vi "信号光谱2.vi"() -> ()   [LabVIEW 2015]
uses:
  <vilib>/Utility/file.llb/Write Delimited Spreadsheet (DBL).vi
  <vilib>/Analysis/NI_AALBase.lvlib
panel:
  out "最终存储路径":path
  in  "停止程序":bool
  in  "上升下降沿/s":dbl format="%.2p"
  in  "延时/s":dbl format="%.2p"
  in  "占空比/%":dbl=3.0 format="%.2p"
  in  "高电平/V":dbl=4.0 format="%.2p"
  in  "频率/Hz":dbl=100.0 format="%.3p"
  in  "低电平/V":dbl min=0.0 max=5.0 format="%.2p"
  out "configure error out":errorcluster
  in  "设置参数":bool
  out "output control error  4":errorcluster
  in  "低电平持续输出":bool
  in  "Output 1":bool
  out "output control error  5":errorcluster
  in  "脉冲作用时间/s":dbl=1.0
  in  "测量高电平/V":dbl=4.0
  out "output control error  2":errorcluster
  in  "测量次数":i32=1
  in  "开始测量":bool
  in  "上升下降沿":i32(ring)=1 items=["上升沿", "下降沿"]
  in  "channel输出口":i32(ring) items=["Channel 1", "Channel 2"]
  in  "输出信号波形":u16(ring) items=["Pulse"]
  out "output control error  3":errorcluster
  out "Output":bool
  in  "VISA 信号发生器":refnum<visa-resource-name>="USB0::0x1AB1::0x0641::DG4E192200870::INSTR"
  out "Spectrum":cluster{"Y":dbl[], "Y":dbl[]}[](graph)
  in  "计数器":dbl=720.0
  out "波长范围":dbl[](array[numeric])
  in  "选项卡控件":enum32{"IHR 550", "CCD"}(tab)
  in  "Move To\nTarget Positions":bool
  out "Current UniqueID":string="Mono4"
  in  "Mono ID":string(combo)="Mono1"
  in  "Connect":bool
  out "Initialized JY":bool=TRUE
  in  "Force\nInitialization":bool
  in  "Target Grating":string(combo)="2"
  out "Current Description":string="1" caption="Description"
  out "Grating Index":i32=1
  out "Current Grating":dbl=1200.0
  out "Units":string="nm"
  out "Current WL":dbl=897.9988
  out "Exit Mirror\nPosition":i32(ring)=2 items=["EntranceMirror", "ExitMirror", "Front", "Side"]
  out "Entrance Mirror\nPosition":i32(ring)=2 items=["EntranceMirror", "ExitMirror", "Front", "Side"]
  out "Units 2":string="mm"
  out "Front Entrance":dbl
  in  "Target WL":dbl=2670.0
  in  "Exit Mirror":u16(ring)=3 caption="Target Position Exit Mirror" items=["Front"=2, "Side"=3]
  in  "Entrance Mirror":u16(ring)=2 caption="Target Position\nEntrance Mirror" items=["Front"=2, "Side"=3]
  in  "Target\nFront Entrance":dbl=1.0
  in  "Commande tab":T1(tab)
  in  "Area Number to Display":i32
  in  "Reformat":bool
  in  "GAIN":u16(ring)=2 caption="Device Name" items=["High Light", "Best Dynamic Range", "High Sensitivity"]
  in  "ADC":u16(ring) caption="Device Name" items=["20 kHz       ", " 1 MHz       ", " 1 MHz Ultra "]
  in  "Number of Areas :":u16=1 min=1 step=1
  in  "Integration time (ms) :":i32=5000
  out "Uniques ID":u16(ring) items=["CCD1", "CCD2"]
  in  "Device Name":u16(ring) items=["Synapse CCD (Lateral)", "Synapse_IGA (Axial)"]
  in  "Signal type :":enum16{"TTL Rising Edge", "TTL Falling Edge"}(ring)=enum."TTL Falling Edge"
  in  "Trigger Type :":u16(ring) items=["On Start"=1, "Per Acquisition"=2]
  in  "trigSigTypeString":string
  in  "trigEventString":string
  in  "Enable InputTriggers :":bool
  in  "Number of Cleans":i32=1
  in  "MultiAcqShutterMode":i32(ring)=3 items=["Open For All Spectra"=1, "Open for Each Spectrum"=3]
  in  "Accumulations:":u16=10 min=1 step=1
  in  "Multi Accumulation mode:":bool
  out "Y Pixels:":i32=256
  out "DataSize":i32=1024
  out "X Pixels:":i32=1024
  out "Firmware\nVersion":string="V1.20 CCD_4000"
  out "initialized ?":bool=TRUE
  in  "Continuous":bool
  in  "CCD Busy":bool
  out "indicator":string="Ready !"
  in  "initialize":bool
  in  "ShutterOpen":bool=TRUE caption="Shutter enable"
  in  "Save Backlight":bool
  in  "Acquire":bool
  in  "Temperature":bool
  in  "Setup":bool
  in  "起始波长":dbl=2406.79
  in  "终止波长":dbl=2919.91
  out "Acq Time(ms)":u32=3401
  in  "Close":bool=TRUE
  out "JYCCDLib.IJYCCDReqd":refnum<k7>
  out "areas :":i32[][](array[numeric])=[[1], [1], [1], [1024], [256], [1], [256]]
  in  "Constante de condition\n(Voir l'aide contextuelle)":bool
  out "temp graph":dbl(graph)=-134.538067
  out "ADC Number":i32[](array[numeric])=[0, 1, 2, 3, 4]
  out "Gain Number":i32[](array[numeric])=[10, 11, 12, 13, 8, 2]
  out "trigAddress":i32
  out "Data":i32[][](graph)
  out "error out":errorcluster
  out "Gratings":dbl[](array[numeric])=[1200.0, 300.0]
  out "Backlight":i32[][](graph)
  out "data 2":i32[][](graph)
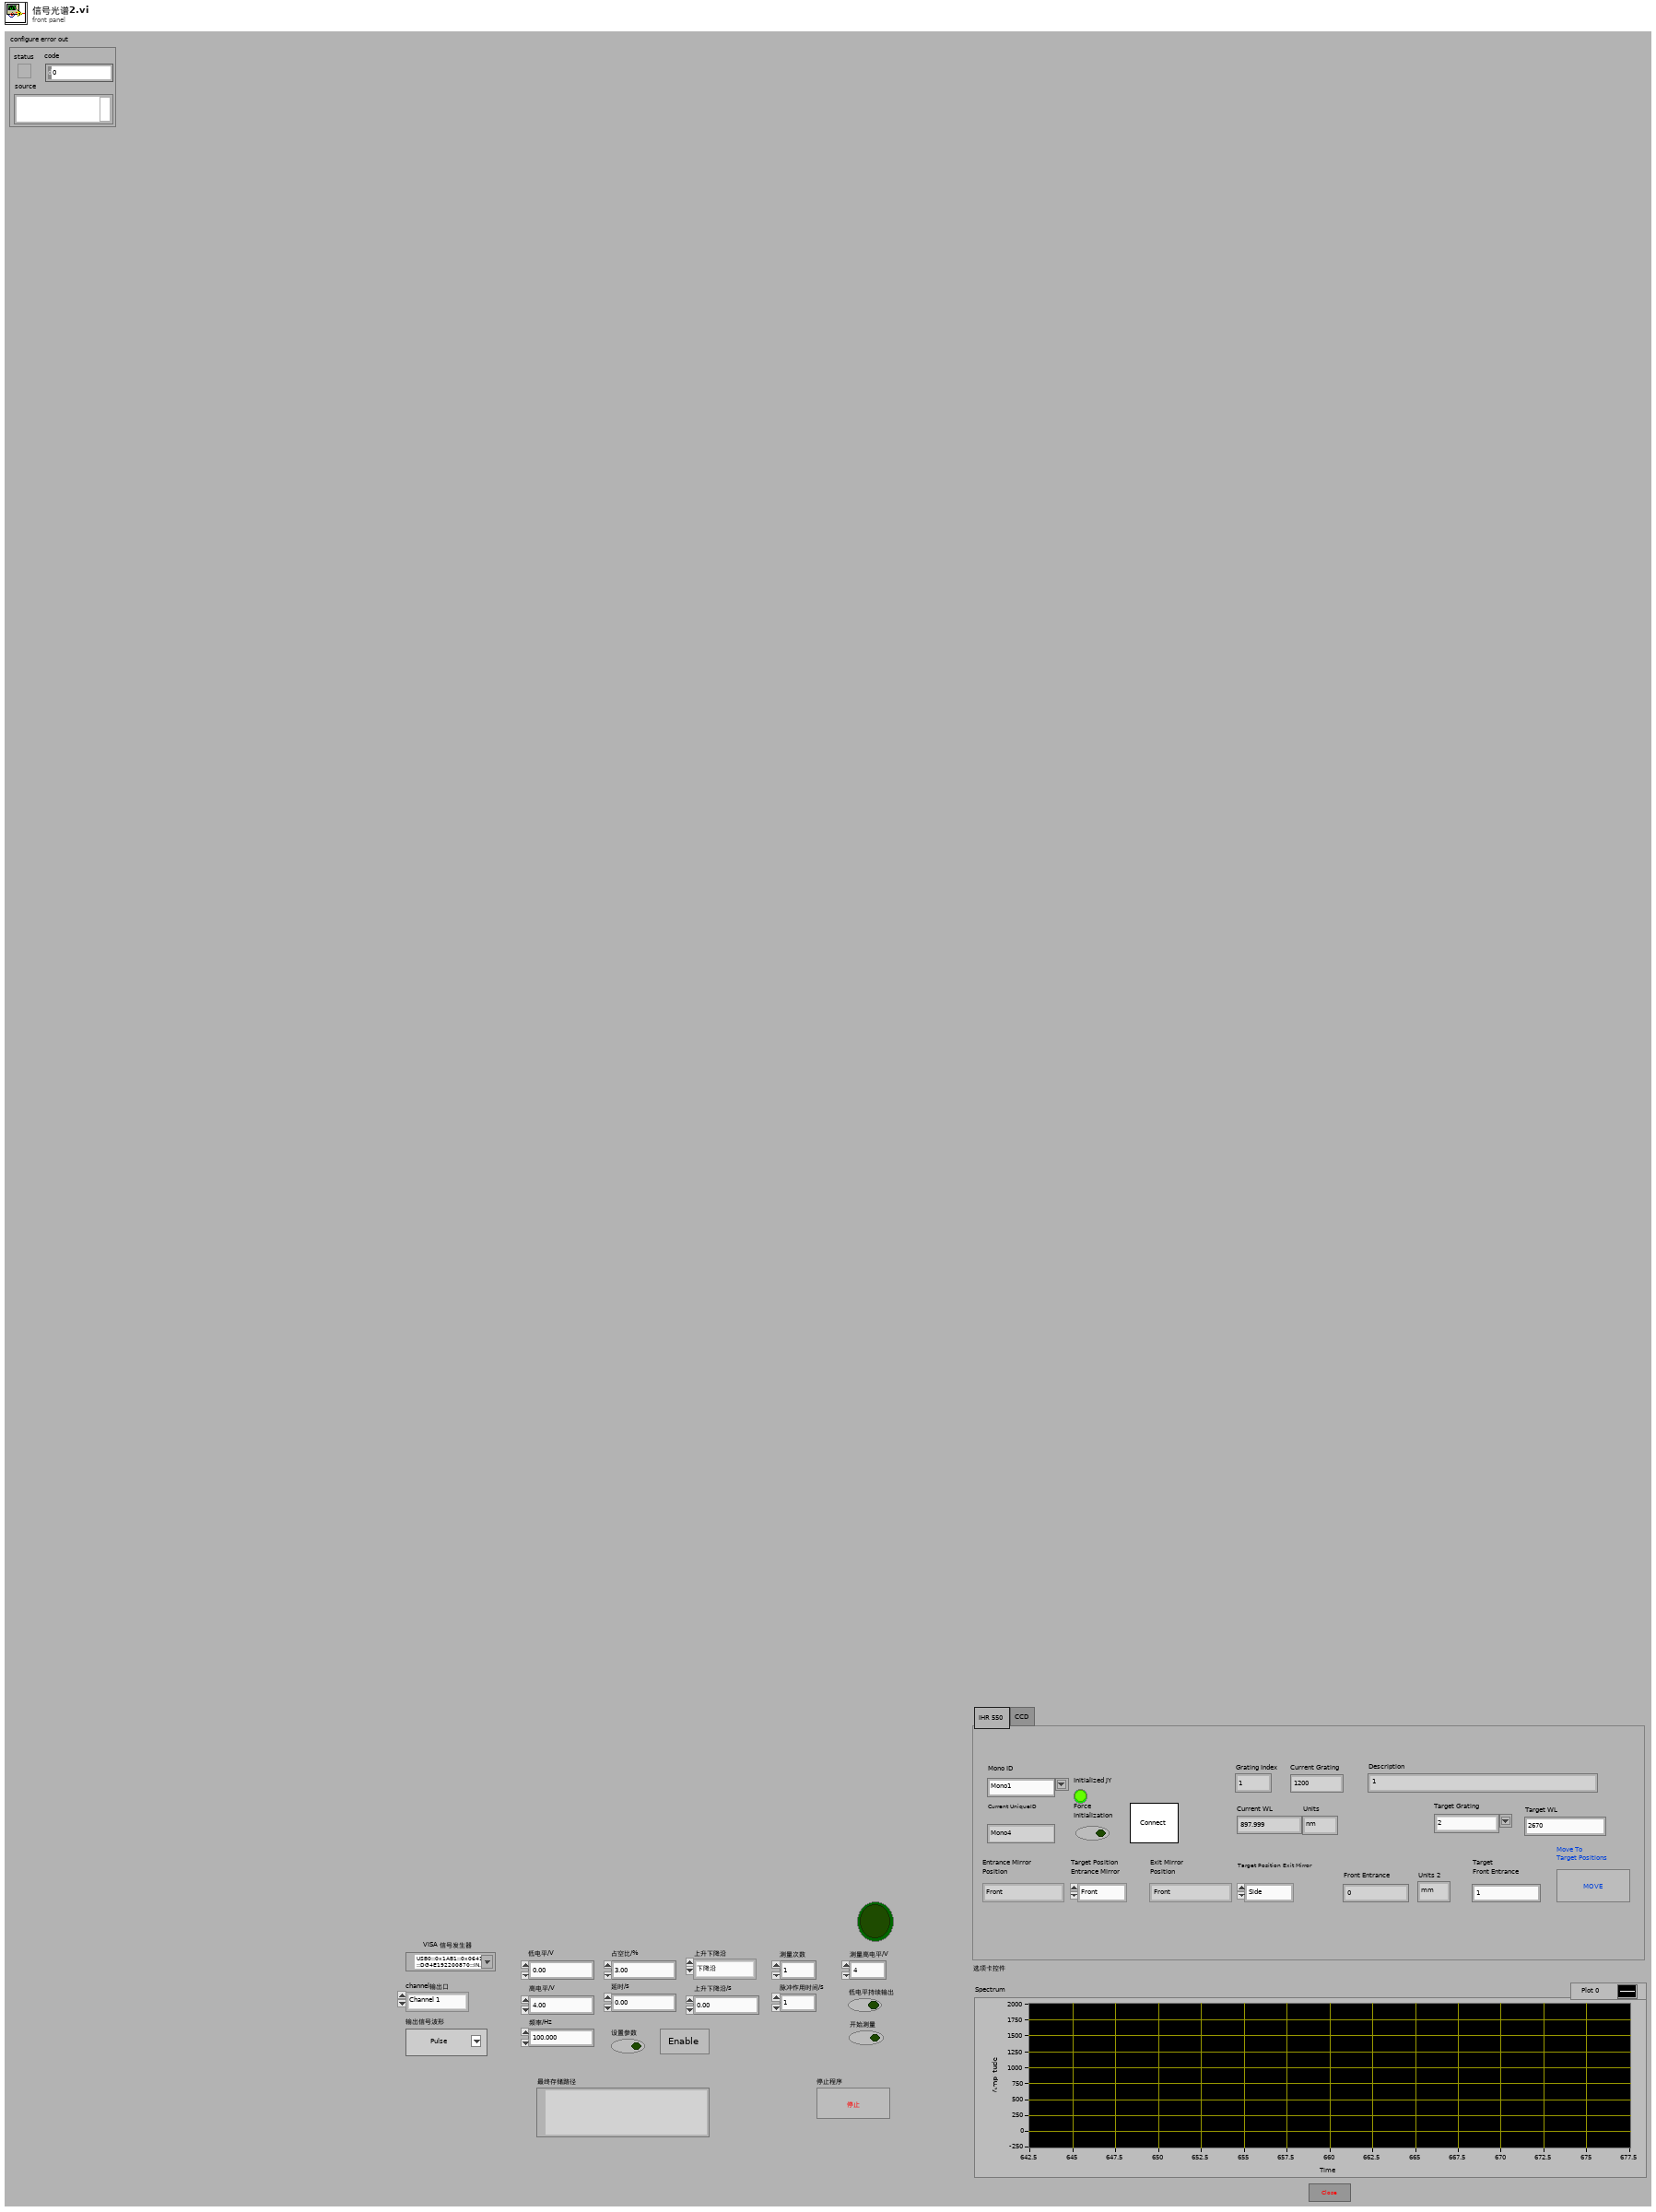
[diagram p1: front panel]
types:
  T1 = enum32{"Settings", "Trigger In", "Multi-Accu.", "Infos"}
  T2 = enum8{"Enabled", "Disabled", "Disabled and Grayed Out"}
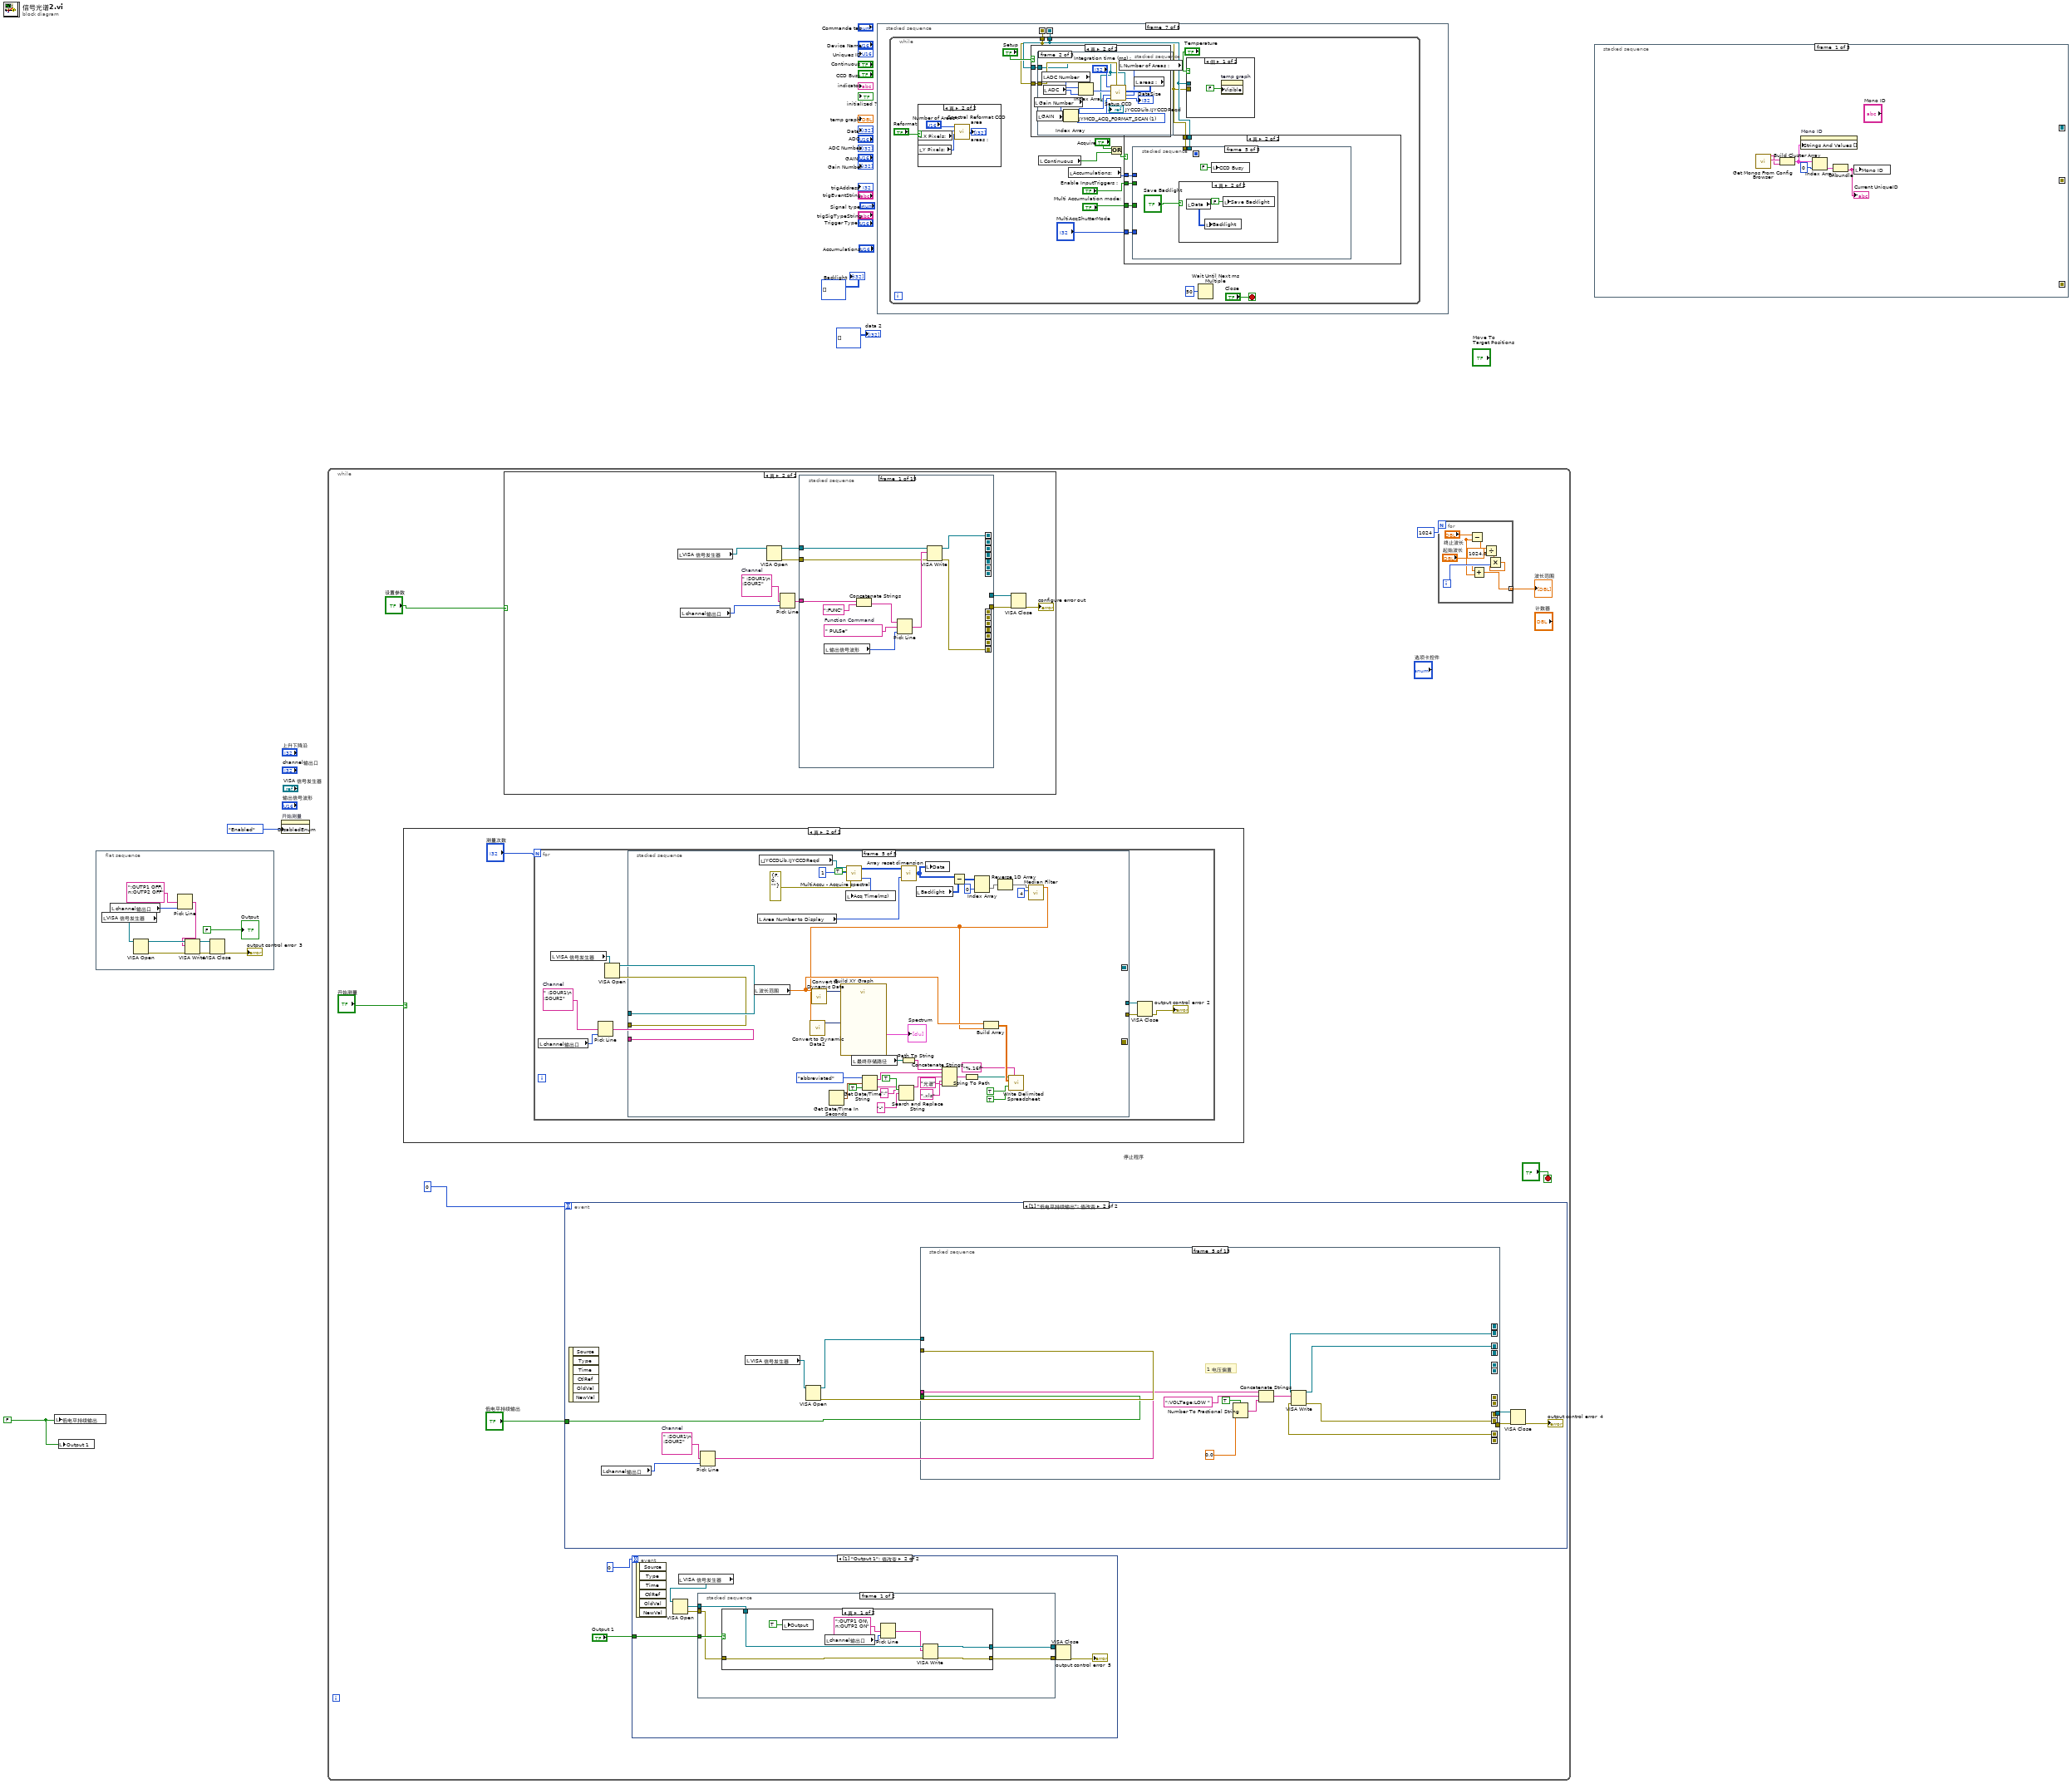
[diagram p0: block diagram]
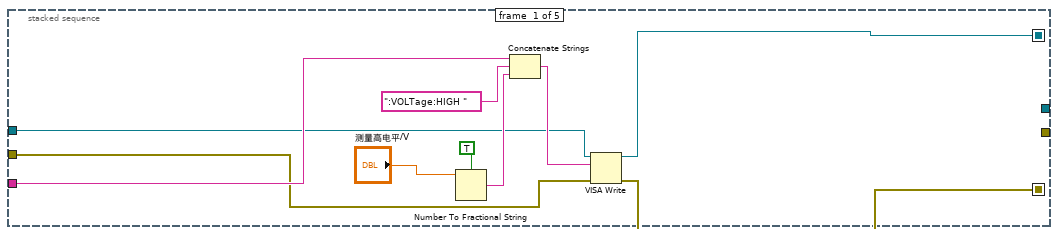
[diagram p3: hidden frame]
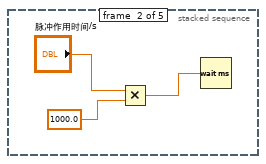
[diagram p4: hidden frame]
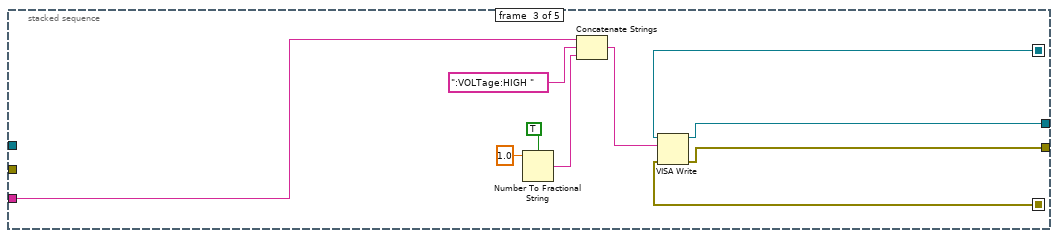
[diagram p5: hidden frame]
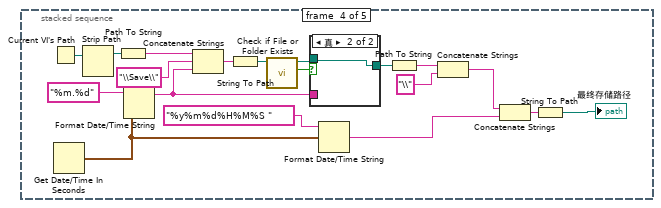
[diagram p6: hidden frame]
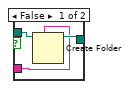
[diagram p7: hidden frame]
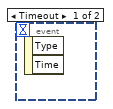
[diagram p8: hidden frame]
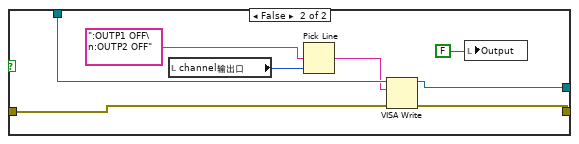
[diagram p9: hidden frame]
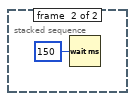
[diagram p10: hidden frame]
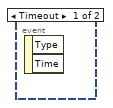
[diagram p11: hidden frame]
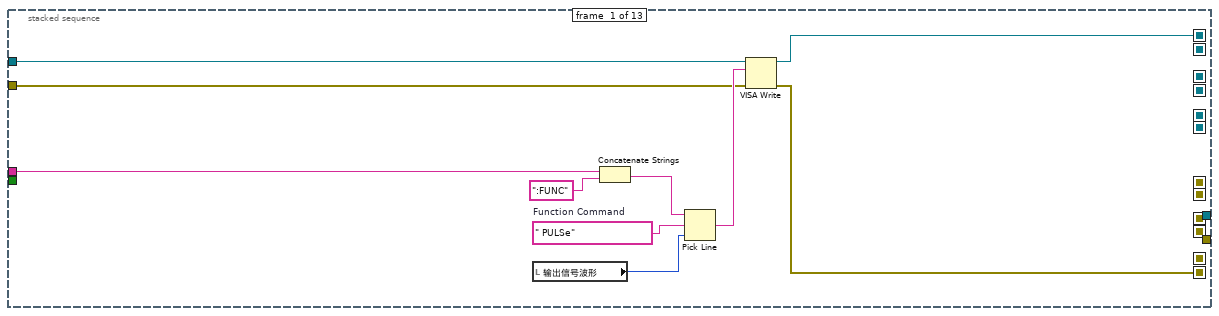
[diagram p12: hidden frame]
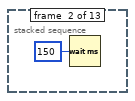
[diagram p13: hidden frame]
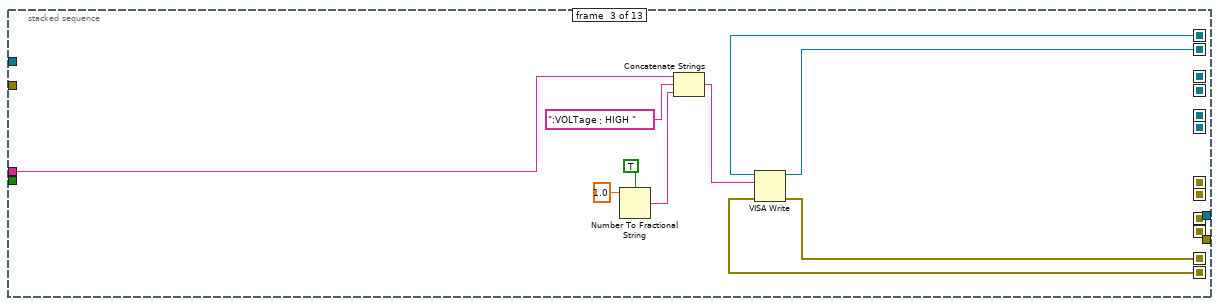
[diagram p14: hidden frame]
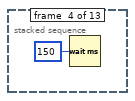
[diagram p15: hidden frame]
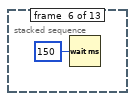
[diagram p16: hidden frame]
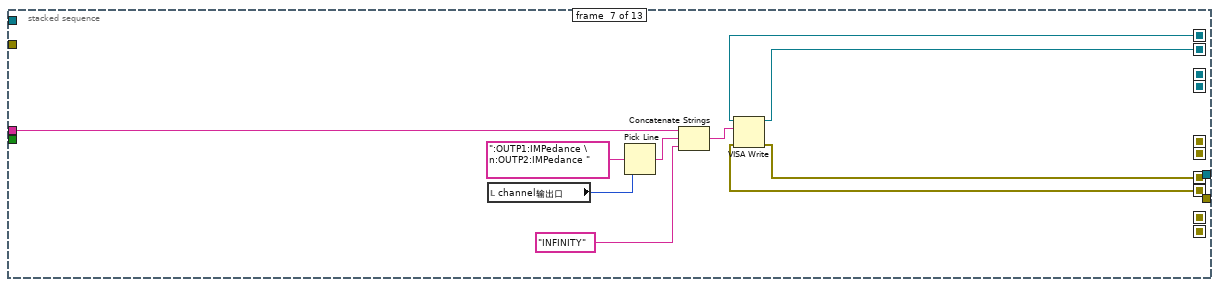
[diagram p17: hidden frame]
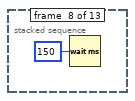
[diagram p18: hidden frame]
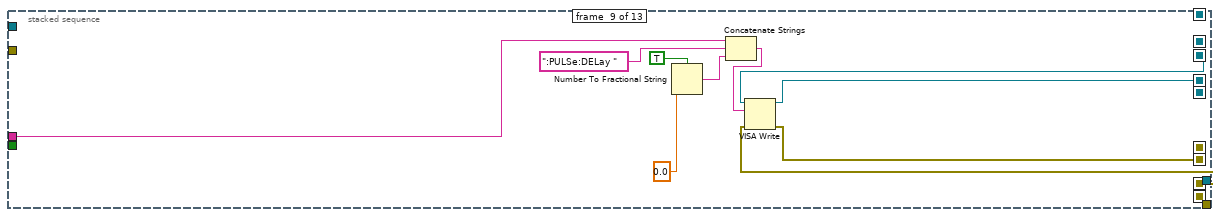
[diagram p19: hidden frame]
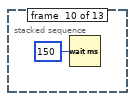
[diagram p20: hidden frame]
diagram:
  w1 = FALSE
  n1 = local write "低电平持续输出"(w1) -> ()
  n2 = local write "Output 1"(w1) -> ()
  n3 = flat-sequence {
    frame #0 {
      n4 = local read "VISA 信号发生器"() -> (w8:refnum<visa-resource-name>)
      n5 = local read "channel输出口"() -> (w6:i32)
      n6 = VISA Open(VISA resource name=w8) -> (VISA resource name=w14:refnum<visa-resource-name>, error out=w13:errorcluster)  [unwired: 4 in]
      n7 = Pick Line(multi-line string=":OUTP1 OFF\n:OUTP2 OFF" ("write buffer"), line index=w6) -> (output string=w5:string)  [unwired: 1 in]
      n8 = VISA Write(VISA resource name=w14, write buffer=w5, error in (no error)=w13) -> (VISA resource name out=w11:refnum<visa-resource-name>, error out=w10:errorcluster)  [unwired: 1 out]
      n9 = VISA Close(VISA resource name=w11, error in (no error)=w10) -> (error out=→"output control error  3":errorcluster)
      "Output" <- FALSE ("布尔")
    }
  }
  n10 = property on="开始测量" class="Bool"("DisabledEnum"=T2."Enabled" ("禁用")) -> ()  [unwired: 2 in, 2 out]
  n11 = while {
    stop <- "停止程序" stop-if-true
    n12 = case shown="真" "开始测量" {
      frame False {
      }
      frame True {
        n13 = for {
          N: "测量次数" -> [_]
          w34 = " :SOUR1\n :SOUR2"  # Channel
          n14 = local read "channel输出口"() -> (w35:i32)
          n15 = local read "VISA 信号发生器"() -> (w41:refnum<visa-resource-name>)
          n16 = Pick Line(multi-line string=w34, line index=w35) -> (output string=w33:string)  [unwired: 1 in]
          n17 = VISA Open(VISA resource name=w41) -> (VISA resource name=w40:refnum<visa-resource-name>, error out=w39:errorcluster)  [unwired: 4 in]
          n18 = stacked-sequence {
            seq-local: [w44 _ _ _ _] -> [_ _ w57 _ _]
            seq-local: [w43 _ _ _ _] -> [_ _ w56 _ _]
            tunnel: w40 -> [w46 _ _ _ _]
            tunnel: w39 -> [w45 _ _ _ _]
            tunnel: [_ _ w59 _ _] -> w38
            tunnel: [_ _ w58 _ _] -> w37
            tunnel: w33 -> [w47 _ w55 _ _]
            frame #0 {
              n19 = Number To Fractional String(use system decimal point (T)=TRUE ("使用系统小数点(T)"), number="测量高电平/V") -> (F-format string=w49:string)  [unwired: 2 in]
              n20 = Concatenate Strings ("连接字符串")(w47, ":VOLTage:HIGH ", w49) -> (w48:string)
              n21 = VISA Write(VISA resource name=w46, write buffer=w48, error in (no error)=w45) -> (VISA resource name out=w44:refnum<visa-resource-name>, error out=w43:errorcluster)  [unwired: 1 out]
            }
            frame #1 {
              n22 = Multiply(x="脉冲作用时间/s", y=1000.0) -> (x*y=w52:dbl)
              n23 = Wait (ms)(milliseconds to wait=w52) -> ()  [unwired: 1 out]
            }
            frame #2 {
              n24 = Number To Fractional String(use system decimal point (T)=TRUE ("使用系统小数点(T)"), number=1.0 ("数字")) -> (F-format string=w62:string)  [unwired: 2 in]
              n25 = Concatenate Strings ("连接字符串")(w55, ":VOLTage:HIGH ", w62) -> (w61:string)
              n26 = VISA Write(VISA resource name=w57, write buffer=w61, error in (no error)=w56) -> (VISA resource name out=w59:refnum<visa-resource-name>, error out=w58:errorcluster)  [unwired: 1 out]
            }
            frame #3 {
              n27 = Current VI's Path() -> (path=w70:path)
              n28 = Get Date/Time In Seconds() -> (seconds since 1Jan1904=w72:timestamp)
              n29 = Strip Path(path=w70) -> (stripped path=w71:path)  [unwired: 1 out]
              n30 = Path To String(path=w71) -> (string=w73:string)
              n31 = Format Date/Time String(time format string (%c)="%m.%d" ("时间格式字符串(%c)"), seconds (now)=w72) -> (date/time string=w79:string)  [unwired: 1 in]
              n32 = Concatenate Strings(w73, "\\Save\\" ("字符串"), w79) -> (w74:string)
              n33 = String To Path(string=w74) -> (path=w75:path)
              n34 = call <vilib>:"Check if File or Folder Exists.vi"("path"=w75) -> ("file or folder exists?"=w76:bool, "dup path"=w78:path)  [unwired: 8 in, 1 out]
              n35 = case shown="真" w76 {
                tunnel: [w86 w87] -> w77
                tunnel: w78 -> [w85 w87]
                tunnel: w79 -> [w84 _]
                frame False {
                  n36 = Create Folder(prompt (Create Folder)=w84, path (use dialog)=w85) -> (created path=w86:path)  [unwired: 1 in, 2 out]
                }
                frame True {
                }
              }
              n37 = Format Date/Time String(time format string (%c)="%y%m%d%H%M%S " ("时间格式字符串(%c)"), seconds (now)=w72) -> (date/time string=w82:string)  [unwired: 1 in]
              n38 = Path To String(path=w77) -> (string=w80:string)
              n39 = Concatenate Strings(w80, "\\" ("字符串")) -> (w81:string)
              n40 = Concatenate Strings(w81, w82) -> (w69:string)
              n41 = String To Path(string=w69) -> (path=→"最终存储路径":path)
            }
            frame #4 {
              n42 = local read "波长范围"() -> (w125:dbl[])
              n43 = local read "Area Number to Display"() -> (w92:i32)
              n44 = local read "JYCCDLib.IJYCCDReqd"() -> (w88:refnum<k7>)
              n45 = call "Convert to Dynamic Data"("Array"=w125) -> ("Dynamic Data Type"=w101:dynamicdata)  [unwired: 3 in]
              n46 = Get Date/Time In Seconds() -> (seconds since 1Jan1904=w106:timestamp)
              n47 = call <userlib>:"MultiAccu - Acquire spectral.vi"("error in"=errorcluster {"status"=FALSE, "code"=0, "source"=""}, "Accumulations:"=u16 1, "ShutterOpen"=TRUE, "JYCCDLib.IJYCCDReqd"=w88) -> ("Acq Time(ms)"=w94:u32, "Array Out"=w93:i32[][][])  [unwired: 1 out]
              n48 = local write "Acq Time(ms)"(w94) -> ()
              n49 = local read "最终存储路径"() -> (w120:path)
              n50 = Get Date/Time String(date format (0)=enum16{"short", "long", "abbreviated"}."abbreviated" ("日期格式(0)"), seconds (now)=w106, want seconds? (F)=TRUE ("需要秒？(F)")) -> (date string=w114:string, time string=w109:string)
              n51 = Search and Replace String(replace all?=TRUE ("替换全部？(F)"), input string=w109, search string=":" ("搜索字符串"), replace string="-" ("替换字符串(\"\")")) -> (result string=w113:string)  [unwired: 4 in, 3 out]
              n52 = call <userlib>:"Array reset dimension.vi"("Area Number"=w92, "Array In"=w93) -> ("Array Out"=w95:i32[][])
              n53 = Path To String(path=w120) -> (string=w103:string)
              n54 = local read "Backlight"() -> (w96:i32[][])
              n55 = local write "Data"(w95) -> ()
              n56 = Concatenate Strings(w103, w114, w113, "光谱" ("字符串"), ".xls" ("字符串")) -> (w118:string)
              n57 = Subtract(x=w95, y=w96) -> (x-y=w97:i32[][])
              n58 = String To Path(string=w118) -> (path=w119:path)
              n59 = Index Array(array=w97, index (row)=0 ("索引 (行)")) -> (element=w121:i32[])  [unwired: 1 in]
              n60 = Reverse 1D Array(array=w121) -> (reversed array=w122:i32[])
              n61 = call <vilib>:"Median Filter.vi"("left rank"=4, "X"=w122) -> ("Filtered X"=w124:dbl[])  [unwired: 8 in, 1 out]
              n62 = call "Convert to Dynamic Data2"("Array"=w124) -> ("Dynamic Data Type"=w100:dynamicdata)  [unwired: 3 in]
              n63 = call "Build XY Graph"("Y Input"=w100, "X Input"=w101) -> ("XY Graph"=→"Spectrum":cluster{"Y":dbl[], "Y":dbl[]}[])  [unwired: 8 in, 1 out]
              n64 = Build Array(w125, w124) -> (w123:dbl[][])
              n65 = call-poly <vilib>:"Write Delimited Spreadsheet.vi"("file path (dialog if empty)"=w119, "format (%.3f)"="%.16f", "2D data"=w123, "append to file? (F)"=TRUE, "transpose? (F)"=TRUE) -> ()  [unwired: 9 in, 2 out]
            }
          }
          n66 = VISA Close(VISA resource name=w38, error in (no error)=w37) -> (error out=→"output control error  2":errorcluster)
        }
      }
    }
    n67 = case shown="真" "设置参数" {
      frame False {
      }
      frame True {
        w260 = " :SOUR1\n :SOUR2"  # Channel
        n68 = local read "VISA 信号发生器"() -> (w256:refnum<visa-resource-name>)
        n69 = local read "channel输出口"() -> (w255:i32)
        n70 = VISA Open(VISA resource name=w256) -> (VISA resource name=w262:refnum<visa-resource-name>, error out=w263:errorcluster)  [unwired: 4 in]
        n71 = Pick Line(multi-line string=w260, line index=w255) -> (output string=w259:string)  [unwired: 1 in]
        n72 = stacked-sequence {
          seq-local: [w268 _ _ _ _ _ _ _ _ _ _ _ _ _ _] -> [_ _ w283 _ _ _ _ _ _ _ _ _ _ _ _]
          seq-local: [w267 _ _ _ _ _ _ _ _ _ _ _ _ _ _] -> [_ _ w282 _ _ _ _ _ _ _ w321 _ _ _ _]
          seq-local: [_ _ w281 _ _ _ _ _ _ _ _ _ _ _ _] -> [_ _ _ _ w292 _ _ _ _ _ _ _ _ _ _]
          seq-local: [_ _ w280 _ _ _ _ _ _ _ _ _ _ _ _] -> [_ _ _ _ w291 _ _ _ _ _ _ _ _ _ _]
          seq-local: [_ _ _ _ w290 _ _ _ _ _ _ _ _ _ _] -> [_ _ _ _ _ _ w298 _ _ _ _ _ _ _ _]
          seq-local: [_ _ _ _ w287 _ _ _ _ _ _ _ _ _ _] -> [_ _ _ _ _ _ w297 _ _ _ _ _ _ _ _]
          seq-local: [_ _ _ _ _ _ w305 _ _ _ _ _ _ _ _] -> [_ _ _ _ _ _ _ _ w316 _ _ _ _ _ _]
          seq-local: [_ _ _ _ _ _ w304 _ _ _ _ _ _ _ _] -> [_ _ _ _ _ _ _ _ w315 _ _ _ _ _ _]
          seq-local: [_ _ _ _ _ _ _ _ w309 _ _ _ _ _ _] -> [_ _ _ _ _ _ _ _ _ _ w322 _ _ _ _]
          seq-local: [_ _ _ _ _ _ _ _ w308 _ _ _ _ _ _] -> [_ _ _ _ _ _ _ _ _ _ _ _ _ _ _]
          seq-local: [_ _ _ _ _ _ _ _ _ _ w318 _ _ _ _] -> [_ _ _ _ _ _ _ _ _ _ _ _ w332 _ _]
          seq-local: [_ _ _ _ _ _ _ _ _ _ w319 _ _ _ _] -> [_ _ _ _ _ _ _ _ _ _ _ _ w331 _ _]
          seq-local: [_ _ _ _ _ _ _ _ _ _ _ _ w330 _ _] -> [_ _ _ _ _ _ _ _ _ _ _ _ _ _ w343]
          seq-local: [_ _ _ _ _ _ _ _ _ _ _ _ w329 _ _] -> [_ _ _ _ _ _ _ _ _ _ _ _ _ _ w342]
          tunnel: w262 -> [w273 _ _ _ _ _ _ _ _ _ _ _ _ _ _]
          tunnel: w263 -> [w266 _ _ _ _ _ _ _ _ _ _ _ _ _ _]
          tunnel: w259 -> [w265 _ w279 _ w286 _ w302 _ w313 _ w323 _ w333 _ w346]
          tunnel: [_ _ _ _ _ _ _ _ _ _ _ _ _ _ w341] -> w258
          tunnel: [_ _ _ _ _ _ _ _ _ _ _ _ _ _ w340] -> w257
          frame #0 {
            w270 = " PULSe"  # Function Command
            n73 = local read "输出信号波形"() -> (w264:u16)
            n74 = Concatenate Strings(w265, ":FUNC" ("string (\"\")")) -> (w271:string)
            n75 = Pick Line(string ("")=w271, multi-line string=w270, line index=w264) -> (output string=w269:string)
            n76 = VISA Write(VISA resource name=w273, write buffer=w269, error in (no error)=w266) -> (VISA resource name out=w268:refnum<visa-resource-name>, error out=w267:errorcluster)  [unwired: 1 out]
          }
          frame #1 {
            n77 = Wait (ms)(milliseconds to wait=u32 150) -> ()  [unwired: 1 out]
          }
          frame #2 {
            n78 = Number To Fractional String(use system decimal point (T)=TRUE ("使用系统小数点(T)"), number="低电平/V") -> (F-format string=w277:string)  [unwired: 2 in]
            n79 = Concatenate Strings ("连接字符串")(w279, ":VOLTage:LOW ", w277) -> (w276:string)
            n80 = VISA Write(VISA resource name=w283, write buffer=w276, error in (no error)=w282) -> (VISA resource name out=w281:refnum<visa-resource-name>, error out=w280:errorcluster)  [unwired: 1 out]
          }
          frame #3 {
            n81 = Wait (ms)(milliseconds to wait=u32 150) -> ()  [unwired: 1 out]
          }
          frame #4 {
            # "1 频率"
            n82 = Concatenate Strings(w286, ":FREQ ") -> (w293:string)
            n83 = Format Into String ("格式化写入字符串")(initial string=w293, "频率/Hz") -> (resulting string=w294:string)  [unwired: 2 in, 1 out]
            n84 = VISA Write(VISA resource name=w292, write buffer=w294, error in (no error)=w291) -> (VISA resource name out=w290:refnum<visa-resource-name>, error out=w287:errorcluster)  [unwired: 1 out]
          }
          frame #5 {
            n85 = Wait (ms)(milliseconds to wait=u32 150) -> ()  [unwired: 1 out]
          }
          frame #6 {
            n86 = Number To Fractional String(use system decimal point (T)=TRUE ("使用系统小数点(T)"), number="高电平/V") -> (F-format string=w299:string)  [unwired: 2 in]
            n87 = Concatenate Strings(w302, ":VOLTage:HIGH ", w299) -> (w301:string)
            n88 = VISA Write(VISA resource name=w298, write buffer=w301, error in (no error)=w297) -> (VISA resource name out=w305:refnum<visa-resource-name>, error out=w304:errorcluster)  [unwired: 1 out]
          }
          frame #7 {
            n89 = Wait (ms)(milliseconds to wait=u32 150) -> ()  [unwired: 1 out]
          }
          frame #8 {
            n90 = local read "channel输出口"() -> (w311:i32)
            n91 = Pick Line(multi-line string=":OUTP1:IMPedance \n:OUTP2:IMPedance " ("write buffer"), line index=w311) -> (output string=w310:string)  [unwired: 1 in]
            n92 = Concatenate Strings ("连接字符串")(w313, w310, "INFINITY") -> (w314:string)
            n93 = VISA Write(VISA resource name=w316, write buffer=w314, error in (no error)=w315) -> (VISA resource name out=w309:refnum<visa-resource-name>, error out=w308:errorcluster)  [unwired: 1 out]
          }
          frame #9 {
            n94 = Wait (ms)(milliseconds to wait=u32 150) -> ()  [unwired: 1 out]
          }
          frame #10 {
            n95 = Number To Fractional String(use system decimal point (T)=TRUE ("使用系统小数点(T)"), number="占空比/%") -> (F-format string=w325:string)  [unwired: 2 in]
            n96 = Concatenate Strings(w323, ":PULSe:DCYCle ", w325) -> (w320:string)
            n97 = VISA Write(VISA resource name=w322, write buffer=w320, error in (no error)=w321) -> (VISA resource name out=w318:refnum<visa-resource-name>, error out=w319:errorcluster)  [unwired: 1 out]
          }
          frame #11 {
            n98 = Wait (ms)(milliseconds to wait=u32 150) -> ()  [unwired: 1 out]
          }
          frame #12 {
            n99 = Number To Fractional String(use system decimal point (T)=TRUE ("使用系统小数点(T)"), number="延时/s") -> (F-format string=w336:string)  [unwired: 2 in]
            n100 = Concatenate Strings(w333, ":PULSe:DELay ", w336) -> (w334:string)
            n101 = VISA Write(VISA resource name=w332, write buffer=w334, error in (no error)=w331) -> (VISA resource name out=w330:refnum<visa-resource-name>, error out=w329:errorcluster)  [unwired: 1 out]
          }
          frame #13 {
            n102 = Wait (ms)(milliseconds to wait=u32 150) -> ()  [unwired: 1 out]
          }
          frame #14 {
            w347 = ":LEADing\n:TRAiling "  # Channel
            w352 = ":PULSe:TRANsition"  # VOLTage:Offset
            n103 = local read "上升下降沿"() -> (w348:i32)
            n104 = Pick Line(multi-line string=w347, line index=w348) -> (output string=w344:string)  [unwired: 1 in]
            n105 = Number To Fractional String(use system decimal point (T)=TRUE ("使用系统小数点(T)"), number="上升下降沿/s") -> (F-format string=w345:string)  [unwired: 2 in]
            n106 = Concatenate Strings(w346, w352, w344, w345) -> (w349:string)
            n107 = VISA Write(VISA resource name=w343, write buffer=w349, error in (no error)=w342) -> (VISA resource name out=w341:refnum<visa-resource-name>, error out=w340:errorcluster)  [unwired: 1 out]
          }
        }
        n108 = VISA Close(VISA resource name=w258, error in (no error)=w257) -> (error out=→"configure error out":errorcluster)
      }
    }
    n109 = event shown="[1] \"低电平持续输出\": 值改变" {
      selector: _ -> [_ _]
      dyn-events: _ -> [_ _]
      timeout: u32 0 ("Time") -> [_ _]
      tunnel: "低电平持续输出" -> [_ w155]
      event Timeout {
        n110 = event-data() -> ()  [unwired: 1 in, 2 out]
      }
      event "低电平持续输出": Value Change {
        w159 = " :SOUR1\n :SOUR2"  # Channel
        n111 = event-data() -> ()  [unwired: 1 in, 6 out]
        n112 = local read "channel输出口"() -> (w160:i32)
        n113 = Pick Line(multi-line string=w159, line index=w160) -> (output string=w158:string)  [unwired: 1 in]
        n114 = local read "VISA 信号发生器"() -> (w163:refnum<visa-resource-name>)
        n115 = VISA Open(VISA resource name=w163) -> (VISA resource name=w162:refnum<visa-resource-name>, error out=w161:errorcluster)  [unwired: 4 in]
        n116 = stacked-sequence {
          seq-local: [w169 _ _ _ _ _ _ _ _ _ _ _ _] -> [_ _ w184 _ _ _ _ _ _ _ _ _ _]
          seq-local: [w168 _ _ _ _ _ _ _ _ _ _ _ _] -> [_ _ w183 _ _ _ _ _ _ _ _ _ _]
          seq-local: [_ _ w182 _ _ _ _ _ _ _ _ _ _] -> [_ _ _ _ w187 _ _ _ _ _ _ _ _]
          seq-local: [_ _ w181 _ _ _ _ _ _ _ _ _ _] -> [_ _ _ _ w188 _ _ _ _ _ _ _ _]
          seq-local: [_ _ _ _ w196 _ _ _ _ _ _ _ _] -> [_ _ _ _ _ _ w207 _ _ _ _ _ _]
          seq-local: [_ _ _ _ w195 _ _ _ _ _ _ _ _] -> [_ _ _ _ _ _ w206 _ _ _ _ _ _]
          seq-local: [_ _ _ _ _ _ w200 _ _ _ _ _ _] -> [_ _ _ _ _ _ _ _ w210 _ _ _ _]
          seq-local: [_ _ _ _ _ _ w199 _ _ _ _ _ _] -> [_ _ _ _ _ _ _ _ w209 _ _ _ _]
          seq-local: [_ _ _ _ _ _ _ _ w213 _ _ _ _] -> [_ _ _ _ _ _ _ _ _ _ w224 _ _]
          seq-local: [_ _ _ _ _ _ _ _ w212 _ _ _ _] -> [_ _ _ _ _ _ _ _ _ _ w223 _ _]
          seq-local: [_ _ _ _ _ _ _ _ _ _ w221 _ _] -> [_ _ _ _ _ _ _ _ _ _ _ _ w238]
          seq-local: [_ _ _ _ _ _ _ _ _ _ w220 _ _] -> [_ _ _ _ _ _ _ _ _ _ _ _ w237]
          tunnel: w162 -> [w174 _ _ _ _ _ _ _ _ _ _ _ _]
          tunnel: w161 -> [w167 _ _ _ _ _ _ _ _ _ _ _ _]
          tunnel: w158 -> [w166 _ w180 _ w193 _ w204 _ w214 _ w227 _ _]
          tunnel: [_ _ _ _ _ _ _ _ _ _ _ _ w236] -> w157
          tunnel: [_ _ _ _ _ _ _ _ _ _ _ _ w234] -> w156
          tunnel: w155 -> [_ _ _ _ _ _ _ _ _ _ _ _ w235]
          frame #0 {
            w171 = " PULSe"  # Function Command
            n117 = local read "输出信号波形"() -> (w165:u16)
            n118 = Concatenate Strings(w166, ":FUNC" ("string (\"\")")) -> (w172:string)
            n119 = Pick Line(string ("")=w172, multi-line string=w171, line index=w165) -> (output string=w170:string)
            n120 = VISA Write(VISA resource name=w174, write buffer=w170, error in (no error)=w167) -> (VISA resource name out=w169:refnum<visa-resource-name>, error out=w168:errorcluster)  [unwired: 1 out]
          }
          frame #1 {
            n121 = Wait (ms)(milliseconds to wait=u32 150) -> ()  [unwired: 1 out]
          }
          frame #2 {
            n122 = Number To Fractional String(use system decimal point (T)=TRUE ("使用系统小数点(T)"), number=1.0 ("数字")) -> (F-format string=w178:string)  [unwired: 2 in]
            n123 = Concatenate Strings ("连接字符串")(w180, ":VOLTage：HIGH ", w178) -> (w177:string)
            n124 = VISA Write(VISA resource name=w184, write buffer=w177, error in (no error)=w183) -> (VISA resource name out=w182:refnum<visa-resource-name>, error out=w181:errorcluster)  [unwired: 1 out]
          }
          frame #3 {
            n125 = Wait (ms)(milliseconds to wait=u32 150) -> ()  [unwired: 1 out]
          }
          frame #4 {
            # "1 电压偏置"
            n126 = Number To Fractional String(use system decimal point (T)=TRUE ("使用系统小数点(T)"), number=0.0 ("数字")) -> (F-format string=w191:string)  [unwired: 2 in]
            n127 = Concatenate Strings(w193, ":VOLTage:LOW ", w191) -> (w192:string)
            n128 = VISA Write(VISA resource name=w187, write buffer=w192, error in (no error)=w188) -> (VISA resource name out=w196:refnum<visa-resource-name>, error out=w195:errorcluster)  [unwired: 1 out]
          }
          frame #5 {
            n129 = Wait (ms)(milliseconds to wait=u32 150) -> ()  [unwired: 1 out]
          }
          frame #6 {
            n130 = local read "channel输出口"() -> (w202:i32)
            n131 = Pick Line(multi-line string=":OUTP1:IMPedance \n:OUTP2:IMPedance " ("write buffer"), line index=w202) -> (output string=w201:string)  [unwired: 1 in]
            n132 = Concatenate Strings ("连接字符串")(w204, w201, "INFINITY") -> (w205:string)
            n133 = VISA Write(VISA resource name=w207, write buffer=w205, error in (no error)=w206) -> (VISA resource name out=w200:refnum<visa-resource-name>, error out=w199:errorcluster)  [unwired: 1 out]
          }
          frame #7 {
            n134 = Wait (ms)(milliseconds to wait=u32 150) -> ()  [unwired: 1 out]
          }
          frame #8 {
            n135 = Number To Fractional String(use system decimal point (T)=TRUE ("使用系统小数点(T)"), number=0.0 ("数字")) -> (F-format string=w217:string)  [unwired: 2 in]
            n136 = Concatenate Strings(w214, ":PULSe:DELay ", w217) -> (w215:string)
            n137 = VISA Write(VISA resource name=w210, write buffer=w215, error in (no error)=w209) -> (VISA resource name out=w213:refnum<visa-resource-name>, error out=w212:errorcluster)  [unwired: 1 out]
          }
          frame #9 {
            n138 = Wait (ms)(milliseconds to wait=u32 150) -> ()  [unwired: 1 out]
          }
          frame #10 {
            w228 = ":LEADing\n:TRAiling "  # Channel
            w232 = ":PULSe:TRANsition"  # VOLTage:Offset
            n139 = local read "上升下降沿"() -> (w229:i32)
            n140 = Pick Line(multi-line string=w228, line index=w229) -> (output string=w225:string)  [unwired: 1 in]
            n141 = Number To Fractional String(use system decimal point (T)=TRUE ("使用系统小数点(T)"), number=0.0 ("数字")) -> (F-format string=w226:string)  [unwired: 2 in]
            n142 = Concatenate Strings(w227, w232, w225, w226) -> (w230:string)
            n143 = VISA Write(VISA resource name=w224, write buffer=w230, error in (no error)=w223) -> (VISA resource name out=w221:refnum<visa-resource-name>, error out=w220:errorcluster)  [unwired: 1 out]
          }
          frame #11 {
            n144 = Wait (ms)(milliseconds to wait=u32 150) -> ()  [unwired: 1 out]
          }
          frame #12 {
            n145 = case shown="假" w235 {
              tunnel: w238 -> [w246 w247]
              tunnel: [w245 w254] -> w234
              tunnel: w237 -> [w244 w252]
              tunnel: [w243 w253] -> w236
              frame True {
                n146 = local write "Output"(TRUE ("布尔")) -> ()
                n147 = local read "channel输出口"() -> (w240:i32)
                n148 = Pick Line(multi-line string=":OUTP1 ON\n:OUTP2 ON" ("write buffer"), line index=w240) -> (output string=w239:string)  [unwired: 1 in]
                n149 = VISA Write(VISA resource name=w246, write buffer=w239, error in (no error)=w244) -> (VISA resource name out=w243:refnum<visa-resource-name>, error out=w245:errorcluster)  [unwired: 1 out]
              }
              frame False {
                n150 = local read "channel输出口"() -> (w249:i32)
                n151 = Pick Line(multi-line string=":OUTP1 OFF\n:OUTP2 OFF" ("write buffer"), line index=w249) -> (output string=w248:string)  [unwired: 1 in]
                n152 = VISA Write(VISA resource name=w247, write buffer=w248, error in (no error)=w252) -> (VISA resource name out=w253:refnum<visa-resource-name>, error out=w254:errorcluster)  [unwired: 1 out]
                n153 = local write "Output"(FALSE ("布尔")) -> ()
              }
            }
          }
        }
        n154 = VISA Close(VISA resource name=w157, error in (no error)=w156) -> (error out=→"output control error  4":errorcluster)
      }
    }
    n155 = event shown="[1] \"Output 1\": 值改变" {
      selector: _ -> [_ _]
      dyn-events: _ -> [_ _]
      timeout: u32 0 ("Time") -> [_ _]
      tunnel: "Output 1" -> [_ w130]
      event Timeout {
        n156 = event-data() -> ()  [unwired: 1 in, 2 out]
      }
      event "Output 1": Value Change {
        n157 = event-data() -> ()  [unwired: 1 in, 6 out]
        n158 = local read "VISA 信号发生器"() -> (w126:refnum<visa-resource-name>)
        n159 = VISA Open(VISA resource name=w126) -> (VISA resource name=w129:refnum<visa-resource-name>, error out=w132:errorcluster)  [unwired: 4 in]
        n160 = stacked-sequence {
          tunnel: w130 -> [w137 _]
          tunnel: w132 -> [w136 _]
          tunnel: w129 -> [w135 _]
          tunnel: [w134 _] -> w128
          tunnel: [w133 _] -> w127
          frame #0 {
            n161 = case shown="真" w137 {
              tunnel: w135 -> [w145 w153]
              tunnel: [w144 w152] -> w133
              tunnel: w136 -> [w143 w150]
              tunnel: [w142 w151] -> w134
              frame True {
                n162 = local write "Output"(TRUE ("布尔")) -> ()
                n163 = local read "channel输出口"() -> (w139:i32)
                n164 = Pick Line(multi-line string=":OUTP1 ON\n:OUTP2 ON" ("write buffer"), line index=w139) -> (output string=w138:string)  [unwired: 1 in]
                n165 = VISA Write(VISA resource name=w145, write buffer=w138, error in (no error)=w143) -> (VISA resource name out=w142:refnum<visa-resource-name>, error out=w144:errorcluster)  [unwired: 1 out]
              }
              frame False {
                n166 = local read "channel输出口"() -> (w147:i32)
                n167 = Pick Line(multi-line string=":OUTP1 OFF\n:OUTP2 OFF" ("write buffer"), line index=w147) -> (output string=w146:string)  [unwired: 1 in]
                n168 = VISA Write(VISA resource name=w153, write buffer=w146, error in (no error)=w150) -> (VISA resource name out=w151:refnum<visa-resource-name>, error out=w152:errorcluster)  [unwired: 1 out]
                n169 = local write "Output"(FALSE ("布尔")) -> ()
              }
            }
          }
          frame #1 {
            n170 = Wait (ms)(milliseconds to wait=u32 150) -> ()  [unwired: 1 out]
          }
        }
        n171 = VISA Close(VISA resource name=w128, error in (no error)=w127) -> (error out=→"output control error  5":errorcluster)
      }
    }
    n172 = for {
      N: 1024 -> [_]
      tunnel: [w28] -> w16 mode=indexing
      i -> [w30]
      n173 = Subtract(x="终止波长", y="起始波长") -> (x-y=w26:dbl)
      n174 = Divide(x=w26, y=1024.0) -> (x/y=w24:dbl)
      n175 = Multiply(x=w24, y=w30) -> (x*y=w29:dbl)
      n176 = Add(x=w29, y="起始波长") -> (x+y=w28:dbl)
    }
    "波长范围" <- w16
  }
  n177 = stacked-sequence {
    seq-local: [_ _ _ w373 _ _ _ _] -> [_ _ _ _ w391 w411 w414 w512]
    seq-local: [_ _ _ w372 _ _ _ _] -> [_ _ _ _ w392 w412 w413 w513]
    frame #0 {
      # "initialize all variables"
      n178 = property on="initialize" class="Bool"("Désactivé"=u8 0) -> ()  [unwired: 2 in, 2 out]
      n179 = property on="Acquire" class="Bool"("Visible"=FALSE) -> ()  [unwired: 2 in, 2 out]
      n180 = property on="Setup" class="Bool"("Visible"=FALSE) -> ()  [unwired: 2 in, 2 out]
      n181 = local write "indicator"("" ("indicator")) -> ()
      n182 = local write "initialized ?"(FALSE ("initialized ?")) -> ()
      n183 = local write "Continuous"(FALSE ("Continuous")) -> ()
      n184 = local write "Close"(FALSE ("Close")) -> ()
      n185 = property on="Device Name" class="Ring (严格)"("Désactivé"=u8 0) -> ()  [unwired: 2 in, 2 out]
      n186 = property on="Continuous" class="Bool (严格)"("Visible"=FALSE) -> ()  [unwired: 2 in, 2 out]
      n187 = local write "Commande tab"(T1."Settings" ("Commande tab")) -> ()
    }
    frame #1 {
      # "Read Uniq ID"
      n188 = stacked-sequence {
        frame #0 {
          n189 = call <userlib>:"read detector uniq-id.vi"() -> ("nbr of components"=w365:i32, "UniqueID"=w364:string[], "Name"=w363:string[])  [unwired: 4 out]
          n190 = for {
            N: w365 -> [_]
            tunnel: w364 -> [w367]
            tunnel: w363 -> [w366]
            n191 = property on="Device Name" class="Ring (严格)"("Chaînes []"=w366) -> ()  [unwired: 2 in, 2 out]
            n192 = property on="Uniques ID" class="Ring (严格)"("Chaînes []"=w367) -> ()  [unwired: 2 in, 2 out]
          }
        }
      }
    }
    frame #2 {
      n193 = while {
        stop <- "initialize" stop-if-true
        n194 = local read "Device Name"() -> (w370:u16)
        n195 = local write "Uniques ID"(w370) -> ()
        n196 = local read "Close"() -> (w368:bool)
        n197 = Stop(stop? (T)=w368) -> ()
        n198 = Wait Until Next ms Multiple(millisecond multiple=u32 100 ("n millisecondes")) -> ()  [unwired: 1 out]
      }
    }
    frame #3 {
      n199 = stacked-sequence {
        tunnel: [_ w380 _ _] -> w373
        tunnel: [_ w379 _ _] -> w372
        frame #0 {
          n200 = local write "indicator"("Initializing ..." ("indicator")) -> ()
        }
        frame #1 {
          n201 = local read "Uniques ID"() -> (w377:u16)
          n202 = property on="Uniques ID" class="Ring (严格)"() -> ("Chaînes []"=w378:string[])  [unwired: 2 in, 2 out]
          n203 = Index Array(array=w378, index=w377) -> (element=w376:string)
          n204 = call <userlib>:"Initialize CCD.vi"("Unique id:"=w376) -> ("activeYPixels"=→"Y Pixels:":i32, "JYCCDLib.IJYCCDReqd"=w379:refnum<k7>, "activeXPixels"=→"X Pixels:":i32, "sortie d'erreur"=w380:errorcluster, "FirmwareVersion"=→"Firmware\nVersion":string)  [unwired: 3 out]
        }
        frame #2 {
          n205 = property on="initialize" class="Bool"("Désactivé"=u8 2) -> ()  [unwired: 2 in, 2 out]
          n206 = property on="Device Name" class="Ring (严格)"("Désactivé"=u8 2) -> ()  [unwired: 2 in, 2 out]
          n207 = local write "Continuous"(FALSE ("Continuous")) -> ()
          n208 = property on="Setup" class="Bool"("Visible"=TRUE) -> ()  [unwired: 2 in, 2 out]
        }
        frame #3 {
          n209 = local write "initialized ?"(TRUE ("initialized ?")) -> ()
          n210 = local write "indicator"("Initialized !" ("indicator")) -> ()
        }
      }
    }
    frame #4 {
      # "Actually not working"
      # "Read ADC and GAIN"
      n211 = case shown="真" "Constante de condition\n(Voir l'aide contextuelle)" {
        tunnel: w392 -> [_ w402]
        tunnel: w391 -> [_ w401]
        frame False {
        }
        frame True {
          # "Read Input supported trigger"
          n212 = call <userlib>:"Trigger - Get Supported Input.vi"("JYCCDLib.IJYCCDReqd"=w402, "Error Input"=w401) -> ("trigAddress"=w396:i32, "eventPtr"=w397:i32, "trigEventString"=w400:string, "trigSigType"=w399:i32, "trigSigTypeString"=w398:string)  [unwired: 4 out]
          n213 = local write "trigSigTypeString"(w398) -> ()
          n214 = local write "trigAddress"(w396) -> ()
          n215 = local write "Trigger Type :"(w397) -> ()
          n216 = local write "trigEventString"(w400) -> ()
          n217 = local write "Signal type :"(w399) -> ()
        }
      }
      n218 = call <userlib>:"Init ADC & Gain.vi"("JYCCDLib.IJYCCDReqd"=w392, "input error"=w391) -> ("ADC Number"=w390:i32[], "ADC description"=w395:string[], "Gain Number"=w393:i32[], "Gain description"=w394:string[])
      n219 = local write "Gain Number"(w393) -> ()
      n220 = local write "ADC Number"(w390) -> ()
      n221 = stacked-sequence {
        tunnel: w395 -> [w403 _]
        tunnel: w394 -> [_ w404]
        frame #0 {
          n222 = property on="ADC" class="Ring (严格)"("Chaînes []"=w403) -> ()  [unwired: 2 in, 2 out]
        }
        frame #1 {
          n223 = property on="GAIN" class="Ring (严格)"("Chaînes []"=w404) -> ()  [unwired: 2 in, 2 out]
        }
      }
    }
    frame #5 {
      # "IS multi Accumulation Supported ?"
      n224 = call <userlib>:"MultiAccu - Is Supported.vi"("Error In"=w411, "JYCCDLib.IJYCCDReqd"=w412) -> ("IsOperatingModeSupported"=w405:bool)  [unwired: 3 out]
      n225 = Select(t=0, s=w405, f=2) -> (s? t:f=w408:i32)
      n226 = Select(t=FALSE, s=w405, f=w405) -> (s? t:f=w407:bool)
      n227 = local write "Multi Accumulation mode:"(w407) -> ()
      n228 = property on="Multi Accumulation mode:" class="Bool (严格)"("Désactivé"=w408) -> ()  [unwired: 2 in, 2 out]
      n229 = property on="Multi Accumulation mode:" class="Bool (严格)"("Désactivé"=w408) -> ()  [unwired: 2 in, 2 out]
    }
    frame #6 {
      n230 = while {
        tunnel: w413 -> [w421]
        tunnel: w414 -> [w420]
        stop <- "Close" stop-if-true
        n231 = case shown="真" "Reformat" {
          frame False {
          }
          frame True {
            n232 = local read "Y Pixels:"() -> (w490:i32)
            n233 = local read "X Pixels:"() -> (w492:i32)
            n234 = call <userlib>:"Spectral Reformat CCD area.vi"("Y Pixels:"=w490, "X Pixels:"=w492, "numAreas"="Number of Areas :") -> ("areas :"=→"areas :":i32[][])  [unwired: 3 out]
          }
        }
        n235 = case shown="真" "Setup" {
          tunnel: w420 -> [_ w495]
          tunnel: w421 -> [_ w494]
          frame False {
          }
          frame True {
            n236 = stacked-sequence {
              tunnel: w495 -> [_ w509 _]
              tunnel: w494 -> [_ w497 _]
              frame #0 {
                n237 = local write "indicator"("Setting up the detector" ("indicator")) -> ()
              }
              frame #1 {
                w507 = 1 items=["JYMCD_ACQ_FORMAT_IMAGE", "JYMCD_ACQ_FORMAT_SCAN"] ("Acquisition type")
                n238 = local read "Gain Number"() -> (w502:i32[])
                n239 = local read "GAIN"() -> (w498:u16)
                n240 = local read "ADC Number"() -> (w503:i32[])
                n241 = local read "ADC"() -> (w499:u16)
                n242 = Index Array(array=w502, index=w498) -> (element=w500:i32)
                n243 = Index Array(array=w503, index=w499) -> (element=w501:i32)
                n244 = local read "Number of Areas :"() -> (w505:u16)
                n245 = local read "areas :"() -> (w506:i32[][])
                n246 = call <userlib>:"Setup CCD.vi"("numAreas"=w505, "areas :"=w506, "JYCCDLib.IJYCCDReqd"=w497, "entrée d'erreur (pas d'erreur)"=w509, "Acquisition type"=w507, "Gain"=w500, "Select ADC"=w501, "Integration time(ms)"="Integration time (ms) :") -> ("DataSize"=→"DataSize":i32)  [unwired: 1 out]
                "JYCCDLib.IJYCCDReqd" <- w497
              }
              frame #2 {
                w510 = TRUE ("Visible")
                n247 = property on="Continuous" class="Bool (严格)"("Visible"=w510) -> ()  [unwired: 2 in, 2 out]
                n248 = property on="Acquire" class="Bool"("Visible"=w510) -> ()  [unwired: 2 in, 2 out]
                n249 = local write "indicator"("Ready !" ("indicator")) -> ()
              }
            }
          }
        }
        n250 = local read "Continuous"() -> (w422:bool)
        n251 = local read "Accumulations:"() -> (w417:u16)
        n252 = Or(x="Acquire", y=w422) -> (x .or. y?=w419:bool)
        n253 = case shown="真" w419 {
          tunnel: w421 -> [_ w434]
          tunnel: w420 -> [_ w433]
          tunnel: "Enable InputTriggers :" -> [_ w432]
          tunnel: "Multi Accumulation mode:" -> [_ w431]
          tunnel: w417 -> [_ w430]
          tunnel: "MultiAcqShutterMode" -> [_ w429]
          frame False {
          }
          frame True {
            n254 = stacked-sequence {
              seq-local: [_ _ w447 _ _] -> [_ _ _ w475 _]
              tunnel: w434 -> [_ w436 w451 w474 _]
              tunnel: w433 -> [_ w437 w450 w473 _]
              tunnel: w432 -> [_ w438 _ _ _]
              tunnel: w431 -> [_ _ w449 _ _]
              tunnel: w430 -> [_ _ w448 _ _]
              tunnel: w429 -> [_ _ w446 _ _]
              frame #0 {
                n255 = local write "CCD Busy"(TRUE ("CCD Busy")) -> ()
              }
              frame #1 {
                n256 = case shown="真" w438 {
                  tunnel: w437 -> [w439 w445]
                  tunnel: w436 -> [w440 w444]
                  frame False {
                    n257 = call <userlib>:"Trigger - Disable.vi"("Error In"=w439, "JYCCDLib.IJYCCDReqd"=w440) -> ()  [unwired: 6 out]
                  }
                  frame True {
                    n258 = local read "Trigger Type :"() -> (w441:u16)
                    n259 = local read "Signal type :"() -> (w442:enum16{"TTL Rising Edge", "TTL Falling Edge"})
                    n260 = local read "trigAddress"() -> (w443:i32)
                    n261 = call <userlib>:"Trigger - Enable.vi"("Error In"=w445, "sigType"=w442, "event"=w441, "trigAddress"=w443, "JYCCDLib.IJYCCDReqd"=w444) -> ()  [unwired: 3 out]
                  }
                }
              }
              frame #2 {
                n262 = case shown="真" w449 {
                  selector: w449 -> [_ w457]
                  tunnel: w451 -> [w454 w460]
                  tunnel: w450 -> [w453 w459]
                  tunnel: w448 -> [_ w458]
                  tunnel: [u16 1 ("Accumulations:") w458] -> w447
                  tunnel: w446 -> [_ w456]
                  frame False {
                    n263 = call <userlib>:"MultiAccu - Disable.vi"("Error In"=w453, "JYCCDLib.IJYCCDReqd"=w454) -> ()  [unwired: 4 out]
                  }
                  frame True {
                    n264 = call <userlib>:"MultiAccu - Configure.vi"("JYCCDLib.IJYCCDReqd"=w460, "Cleans Before"="Number of Cleans", "Accumulations:"=w458, "MultiAcqHardwareMode"=w457, "MultiAcqShutterMode"=w456, "Error In"=w459) -> ()  [unwired: 1 in, 9 out]
                  }
                }
              }
              frame #3 {
                n265 = call <userlib>:"MultiAccu - Acquire spectral.vi"("error in"=w473, "Accumulations:"=w475, "ShutterOpen"="ShutterOpen", "JYCCDLib.IJYCCDReqd"=w474) -> ("Acq Time(ms)"=→"Acq Time(ms)":u32, "Array Out"=w472:i32[][][])  [unwired: 1 out]
                n266 = call <userlib>:"Array reset dimension.vi"("Area Number"="Area Number to Display", "Array In"=w472) -> ("Array Out"=w470:i32[][])
                n267 = local read "Backlight"() -> (w469:i32[][])
                n268 = Subtract(x=w470, y=w469) -> (x-y=w467:i32[][])
                n269 = local write "Data"(w470) -> ()
                n270 = local write "data 2"(w467) -> ()
                n271 = Index Array(array=w467, index (row)=0 ("禁用的索引 (列)")) -> (element=w462:i32[])  [unwired: 1 in]
                n272 = local read "波长范围"() -> (w463:dbl[])
                n273 = Reverse 1D Array(array=w462) -> (reversed array=w461:i32[])
                n274 = call "转换至动态数据2"("Array"=w463) -> ("Dynamic Data Type"=w465:dynamicdata)  [unwired: 3 in]
                n275 = call "转换至动态数据"("Array"=w461) -> ("Dynamic Data Type"=w466:dynamicdata)  [unwired: 3 in]
                n276 = call "Build XY Graph2"("Y Input"=w466, "X Input"=w465) -> ("XY Graph"=w464:cluster{"Y":dbl[], "Y":dbl[]}[])  [unwired: 8 in, 1 out]
                n277 = local write "Spectrum"(w464) -> ()
              }
              frame #4 {
                n278 = case shown="真" "Save Backlight" {
                  frame False {
                  }
                  frame True {
                    n279 = local read "Data"() -> (w481:i32[][])
                    n280 = local write "Backlight"(w481) -> ()
                    n281 = local write "Save Backlight"(FALSE ("Save Backlight")) -> ()
                  }
                }
                n282 = local write "CCD Busy"(FALSE ("CCD Busy")) -> ()
              }
            }
          }
        }
        n283 = case shown="假" "Temperature" {
          tunnel: w421 -> [_ w484]
          tunnel: w420 -> [_ w483]
          frame False {
            n284 = property on="temp graph" class="WFChart (严格)"("Visible"=FALSE) -> ()  [unwired: 2 in, 2 out]
          }
          frame True {
            n285 = stacked-sequence {
              tunnel: w484 -> [_ w489]
              tunnel: w483 -> [_ w488]
              frame #0 {
                n286 = property on="temp graph" class="WFChart (严格)"("Visible"=TRUE) -> ()  [unwired: 2 in, 2 out]
              }
              frame #1 {
                w487 = u16 0 items=["° Celsius", "Kelvin", "° Farenheit"] ("units")
                n287 = call <userlib>:"read temperature.vi"("entrée d'erreur (pas d'erreur)"=w488, "units"=w487, "JYCCDLib.IJYCCDReqd"=w489) -> ("Current Temperature"=w486:dbl)
                n288 = local write "temp graph"(w486) -> ()
              }
            }
          }
        }
        n289 = Wait Until Next ms Multiple(millisecond multiple=u32 50 ("n millisecondes")) -> ()  [unwired: 1 out]
      }
    }
    frame #7 {
      n290 = Close Reference(reference=w513, error in (no error)=w512) -> ()  [unwired: 1 out]
    }
  }
  n291 = stacked-sequence {
    seq-local: [_ _ w523 _ _] -> [_ _ _ w533 w538]
    seq-local: [_ _ w522 _ _] -> [_ _ _ w532 _]
    seq-local: [_ _ _ w531 _] -> [_ _ _ _ _]
    frame #0 {
      n292 = call <userlib>:"Get Monos From Config Browser.vi"() -> ("UniqueIDs"=w518:string[], "Mono ID"=w519:string[])  [unwired: 3 in, 1 out]
      n293 = Build Cluster Array(w519, w518) -> (w516:cluster{"String":string, "String":string}[])
      n294 = property on="Mono ID" class="CmbBox"("Strings And Values []"=w516) -> ()  [unwired: 2 in, 2 out]
      n295 = Index Array(array=w516, index=0) -> (element=w517:cluster{"String":string, "String":string})
      n296 = Unbundle(w517) -> ("String"=w514:string)  [unwired: 1 out]
      "Current UniqueID" <- w514
      n297 = local write "Mono ID"(w514) -> ()
    }
    frame #1 {
      n298 = while {
        stop <- "Connect" stop-if-true
        n299 = local read "Mono ID"() -> (w520:string)
        n300 = local write "Current UniqueID"(w520) -> ()
      }
    }
    frame #2 {
      n301 = local read "Mono ID"() -> (w525:string)
      n302 = call <userlib>:"JYInitMono.vi"("Unique ID"=w525, "Force Init"="Force\nInitialization") -> ("Refnum out"=w523:refnum<k7>, "Initialized"=→"Initialized JY":bool, "error out"=w522:errorcluster)  [unwired: 9 in, 2 out]
    }
    frame #3 {
      n303 = call <userlib>:"Show Current Grating.vi"("Refnum in"=w533, "error in (no error)"=w532) -> ("Gratings"=w534:dbl[], "Grating Index"=w528:i32, "Current Grating"=w530:dbl, "Current Description"=w527:string, "error out"=w531:errorcluster)  [unwired: 5 in, 4 out]
      "Gratings" <- w534
      n304 = local write "Current Grating"(w530) -> ()
      n305 = local write "Current Description"(w527) -> ()
      n306 = Number To Decimal String(number=w534) -> (decimal integer string=w536:string[])  [unwired: 1 in]
      n307 = Number To Decimal String(number=w528) -> (decimal integer string=w529:string)  [unwired: 1 in]
      n308 = property on="Target Grating" class="CmbBox"("Value"=w529) -> ()  [unwired: 2 in, 2 out]
      n309 = Build Cluster Array(w536, string[] ["1", "2", "3"]) -> (w537:cluster{"Numeric":string, string}[])
      n310 = property on="Target Grating" class="CmbBox"("Strings And Values []"=w537) -> ()  [unwired: 2 in, 2 out]
    }
    frame #4 {
      n311 = while {
        tunnel: w538 -> [w540]
        stop <- w539 stop-if-true
        n312 = stacked-sequence {
          seq-local: [w544 _ _ _ _] -> [_ w551 w562 _ w569]
          seq-local: [w543 _ _ _ _] -> [_ w550 w561 _ _]
          seq-local: [_ w549 _ _ _] -> [_ _ _ _ _]
          seq-local: [_ w548 _ _ _] -> [_ _ _ _ _]
          seq-local: [_ _ w554 _ _] -> [_ _ _ _ _]
          seq-local: [_ _ w553 _ _] -> [_ _ _ w564 _]
          tunnel: w540 -> [w542 _ _ w565 _]
          frame #0 {
            n313 = call <userlib>:"Show Current Grating.vi"("Refnum in"=w542) -> ("Grating Index"=→"Grating Index":i32, "Current Grating"=→"Current Grating":dbl, "Current Description"=→"Current Description":string, "error out"=w543:errorcluster, "JYMONOLib.IJYMonoReqd"=w544:refnum<k7>)  [unwired: 6 in, 4 out]
          }
          frame #1 {
            n314 = call <userlib>:"JYGetCurrentWL.vi"("error in (no error)"=w550, "JYMONOLib.IJYMonoReqd"=w551) -> ("error out"=w548:errorcluster, "Units"=→"Units":string, "Current WL"=→"Current WL":dbl, "JYMONOLib.IJYMonoReqd 2"=w549:refnum<k7>)  [unwired: 6 in]
          }
          frame #2 {
            w559 = u16 1 items=["Entrance", "Exit"] ("Mirror Number")
            w560 = u16 0 items=["Entrance", "Exit"] ("Mirror Number")
            n315 = call <userlib>:"JYGetMirrorPos.vi"("error in (no error)"=w561, "Mirror"=w560, "Refnum In"=w562) -> ("error out"=w557:errorcluster, "Current Mirror Position"=→"Entrance Mirror\nPosition":i32, "Refnum Out"=w558:refnum<k7>)  [unwired: 1 in]
            n316 = call <userlib>:"JYGetMirrorPos.vi"("error in (no error)"=w557, "Mirror"=w559, "Refnum In"=w558) -> ("error out"=w553:errorcluster, "Current Mirror Position"=→"Exit Mirror\nPosition":i32, "Refnum Out"=w554:refnum<k7>)  [unwired: 1 in]
          }
          frame #3 {
            w567 = u16 0 items=["Front Entrance", "Side Entrance", "Front Exit", "Side Exit", "First Intermediate", "Second Intermediate"] ("Slit")
            n317 = call <userlib>:"JYGetSlits.vi"("MonoRefNum IN"=w565, "Slit"=w567, "error in (no error)"=w564) -> ("Units"=→"Units 2":string, "Slit Width"=→"Front Entrance":dbl, "error out"=→"error out":errorcluster)  [unwired: 13 in, 1 out]
          }
          frame #4 {
            n318 = local read "Move To\nTarget Positions"() -> (w570:bool)
            n319 = case shown="真" w570 {
              tunnel: w569 -> [_ w571]
              frame False {
              }
              frame True {
                n320 = stacked-sequence {
                  seq-local: [w573 _ _ _] -> [_ w579 _ _]
                  seq-local: [_ w577 _ _] -> [_ _ w594 _]
                  seq-local: [_ _ w581 _] -> [_ _ _ w600]
                  seq-local: [_ _ _ w597] -> [_ _ _ _]
                  tunnel: w571 -> [w575 w578 w592 w601]
                  frame #0 {
                    n321 = property on="Target Grating" class="CmbBox"() -> ("Value"=w572:string)  [unwired: 2 in, 2 out]
                    n322 = local read "error out"() -> (w574:errorcluster)
                    n323 = Decimal String To Number(string=w572) -> (number=w576:i32)  [unwired: 2 in, 1 out]
                    n324 = call <userlib>:"JYTurret.vi"("error in (no error)"=w574, "Grating Index"=w576, "JYMONOLib.IJYMonoReqd"=w575) -> ("error out"=w573:errorcluster)  [unwired: 2 out]
                  }
                  frame #1 {
                    # "Move Grating to Target Position"
                    n325 = call <userlib>:"JYMoveToWavelength.vi"("error in (no error)"=w579, "Target WL"="Target WL", "RefNum In"=w578) -> ("error out"=w577:errorcluster)  [unwired: 1 in, 2 out]
                  }
                  frame #2 {
                    w587 = u16 1 items=["Entrance", "Exit"] ("Mirror Number")
                    w586 = u16 0 items=["Entrance", "Exit"] ("Mirror Number")
                    w593 = u16 1 items=["Entrance", "Exit", "Front", "Side"] ("Mirror Number")
                    w596 = u16 0 items=["Entrance", "Exit", "Front", "Side"] ("Mirror Number")
                    # "Move Mirrors"
                    n326 = call <userlib>:"JYMirrorMove.vi"("error in (no error)"=w594, "Mirror Position"="Entrance Mirror", "Mirror Number"=w596, "RefNum In"=w592) -> ("error out"=w591:errorcluster)  [unwired: 6 in, 1 out]
                    n327 = call <userlib>:"JYMirrorMove.vi"("error in (no error)"=w591, "Mirror Position"="Exit Mirror", "Mirror Number"=w593, "RefNum In"=w592) -> ("error out"=w584:errorcluster, "MonoRefNum Out"=w585:refnum<k7>)  [unwired: 6 in]
                    n328 = call <userlib>:"JYGetMirrorPos.vi"("error in (no error)"=w584, "Mirror"=w586, "Refnum In"=w585) -> ("error out"=w589:errorcluster, "Current Mirror Position"=w583:i32, "Refnum Out"=w588:refnum<k7>)  [unwired: 1 in]
                    n329 = local write "Entrance Mirror\nPosition"(w583) -> ()
                    n330 = call <userlib>:"JYGetMirrorPos.vi"("error in (no error)"=w589, "Mirror"=w587, "Refnum In"=w588) -> ("error out"=w581:errorcluster, "Current Mirror Position"=w582:i32)  [unwired: 1 in, 1 out]
                    n331 = local write "Exit Mirror\nPosition"(w582) -> ()
                  }
                  frame #3 {
                    w599 = u16 0 items=["Front Entrance", "Side Entrance", "Front Exit", "Side Exit", "First Intermediate", "Second Intermediate"] ("Slit")
                    # "Set New Slit Positions"
                    n332 = call <userlib>:"JYSlits.vi"("JYMONOLib.IJYMonoReqd"=w601, "Slit"=w599, "error in (no error)"=w600, "Slit Width"="Target\nFront Entrance") -> ("error out"=w597:errorcluster)  [unwired: 1 in, 1 out]
                  }
                }
              }
            }
          }
        }
        n333 = local read "Close"() -> (w539:bool)
      }
    }
  }
  "Backlight" <- i32[][] [] ("Backlight")
  "data 2" <- i32[][] [] ("data 2")
